vi "Update and Acknowledge InterruptBit HW.vi"(5 "Acknowledge?(True)":bool=TRUE, 7 "AcknPeriode":dbl, 8 "error in (no error)":errorcluster, 9 "current time":timestamp, 10 "InterruptBits":i32, 11 "BME_DG_Chnl in":refnum<class "BME_DG_Chnl.lvclass">) -> (0 "error out":errorcluster, 1 "ShotPeriode":dbl, 2 "ChnlBit":bool, 3 "BME_DG_Chnl out":refnum<class "BME_DG_Chnl.lvclass">)   [LabVIEW 2009, in "POLARIS BME DG.lvlib" / "BME_DG_Chnl.lvclass"]
uses:
  BME_DG_Chnl.lvclass
  BME_DG_Chnl.lvclass/BME_DG_Chnl.ctl
  POLARIS BME DG.lvlib
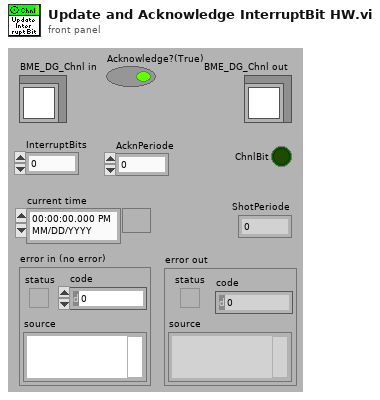
[diagram p1: front panel]
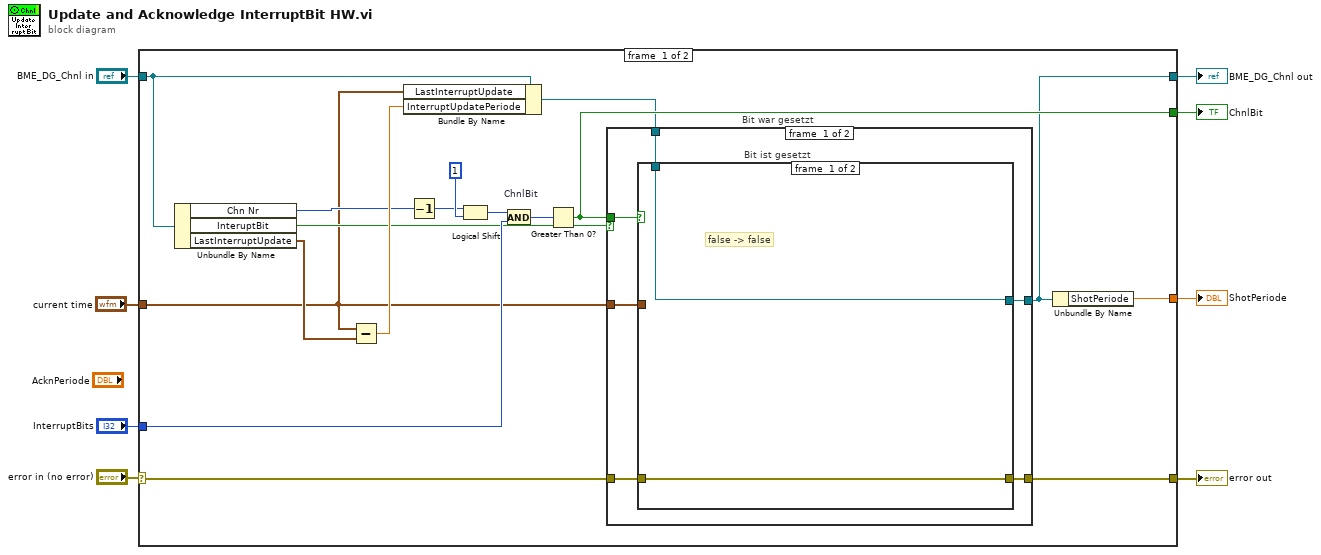
[diagram p0: block diagram]
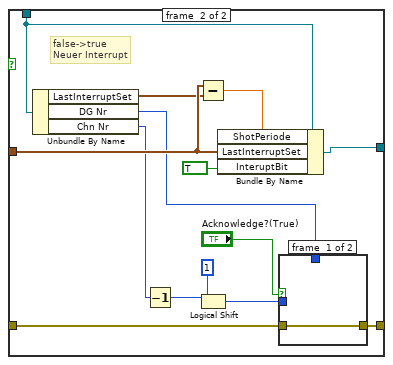
[diagram p2: hidden frame]
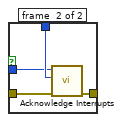
[diagram p3: hidden frame]
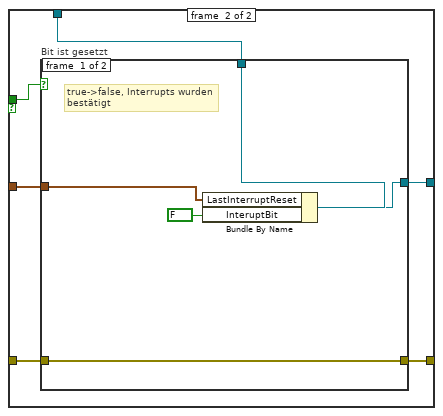
[diagram p4: hidden frame]
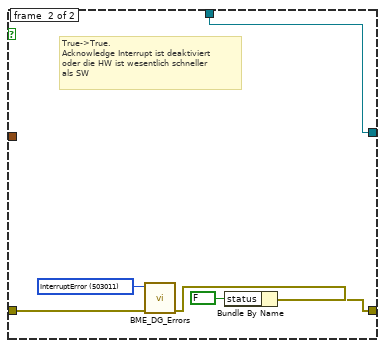
[diagram p5: hidden frame]
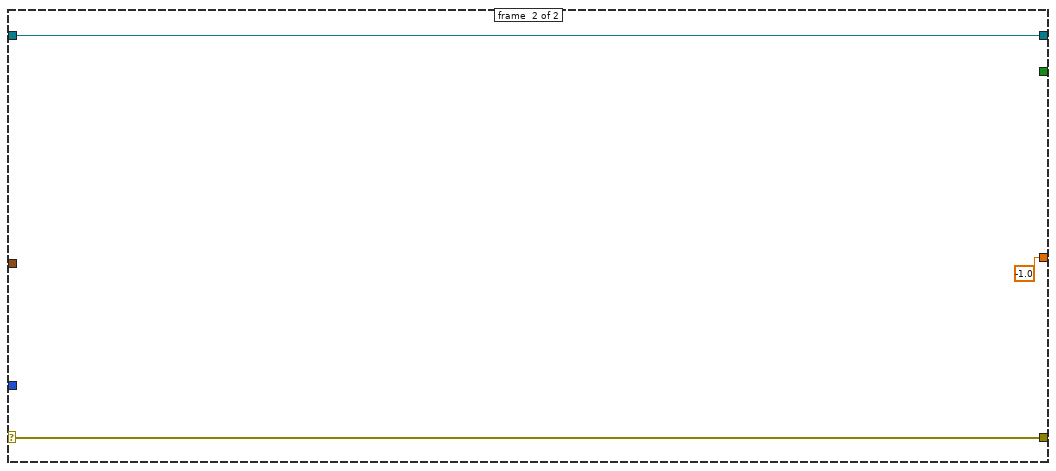
[diagram p6: hidden frame]
diagram:
  n1 = case shown="No Error" "error in (no error)" {
    selector: "error in (no error)" -> [w15 w70]
    tunnel: "BME_DG_Chnl in" -> [w13 w72]
    tunnel: "InterruptBits" -> [w22 _]
    tunnel: [w16 _] -> w6
    tunnel: [w11 w72] -> w5
    tunnel: "current time" -> [w12 _]
    tunnel: [w10 -1.0 ("f")] -> w3
    tunnel: [w14 w70] -> w1
    frame #0 {
      n2 = Unbundle By Name(w13) -> ("Chn Nr"=w18:i32, "InteruptBit"=w17:bool, "LastInterruptUpdate"=w20:timestamp)
      n3 = Subtract(x=w12, y=w20) -> (x-y=w19:dbl)
      n4 = Bundle By Name(cluster=w13, "LastInterruptUpdate"=w12, "InterruptUpdatePeriode"=w19) -> (w9:refnum<class "BME_DG_Chnl.lvclass">)
      n5 = Decrement(x=w18) -> (x-1=w24:i32)
      n6 = Logical Shift(y=w24, x=1) -> (x << y=w23:i32)
      n7 = And "ChnlBit"(x=w23, y=w22) -> (x .and. y?=w21:i32)
      n8 = Greater Than 0?(x=w21) -> (x > 0?=w16:bool)
      n9 = case "Bit war gesetzt" shown="False" w17 {
        tunnel: w16 -> [w31 w58]
        tunnel: w15 -> [w26 w57]
        tunnel: [w27 w56] -> w14
        tunnel: w9 -> [w30 w55]
        tunnel: w12 -> [w28 w54]
        tunnel: [w29 w53] -> w11
        frame #0 {
          n10 = case "Bit ist gesetzt" shown="True" w31 {
            tunnel: w30 -> [w33 w45]
            tunnel: [w33 w47] -> w29
            tunnel: w28 -> [_ w44]
            tunnel: [w32 w37] -> w27
            tunnel: w26 -> [w32 w38]
            frame #0 {
              # "false -> false"
            }
            frame #1 {
              # "false->true \nNeuer Interrupt"
              n11 = Unbundle By Name(w45) -> ("LastInterruptSet"=w43:timestamp, "DG Nr"=w36:i32, "Chn Nr"=w40:i32)
              n12 = Decrement(x=w40) -> (x-1=w41:i32)
              n13 = Subtract(x=w44, y=w43) -> (x-y=w42:dbl)
              n14 = Logical Shift(y=w41, x=1) -> (x << y=w35:i32)
              n15 = Bundle By Name(cluster=w45, "ShotPeriode"=w42, "LastInterruptSet"=w44, "InteruptBit"=TRUE) -> (w47:refnum<class "BME_DG_Chnl.lvclass">)
              n16 = case shown="True" "Acknowledge?(True)" {
                tunnel: w38 -> [w48 w52]
                tunnel: [w48 w51] -> w37
                tunnel: w36 -> [_ w50]
                tunnel: w35 -> [_ w49]
                frame #0 {
                }
                frame #1 {
                  n17 = call "Acknowledge Interrupts.vi"("error in (no error)"=w52, "DG Number"=w50, "Interrupt Ack"=w49) -> ("error out"=w51:errorcluster)  [unwired: 8 in]
                }
              }
            }
          }
        }
        frame #1 {
          n18 = case "Bit ist gesetzt" shown="False" w58 {
            tunnel: w57 -> [w59 w68]
            tunnel: [w59 w65] -> w56
            tunnel: w55 -> [w63 w64]
            tunnel: w54 -> [w61 _]
            tunnel: [w62 w64] -> w53
            frame #0 {
              # "true->false, Interrupts wurden\nbestätigt"
              n19 = Bundle By Name(cluster=w63, "LastInterruptReset"=w61, "InteruptBit"=FALSE) -> (w62:refnum<class "BME_DG_Chnl.lvclass">)
            }
            frame #1 {
              w69 = 503011 items=["Channel refers itself"=503001, "Deadloop"=503002, "Negative Delay"=503003, "Delay Card not found"=503004, "Channel not found"=503005, "Parse Error"=503006, "Not Supported"=503007, "Systen not found"=503008, "To much masters"=503009, "None master in Syterm"=503010, "InterruptError"=503011, "ChnlPeriodeWarning"=503012] ("error")
              # "True->True. \nAcknowledge Interrupt ist deaktiviert\noder die HW ist wesentlich schneller\nals SW"
              n20 = call "BME_DG_Errors.vi"("error in (no error)"=w68, "error"=w69) -> ("error out"=w67:errorcluster)  [unwired: 9 in]
              n21 = Bundle By Name(cluster=w67, "status"=FALSE) -> (w65:errorcluster)
            }
          }
        }
      }
      n22 = Unbundle By Name(w11) -> ("ShotPeriode"=w10:dbl)
    }
    frame #1 {
    }
  }
  "error out" <- w1
  "BME_DG_Chnl out" <- w5
  "ChnlBit" <- w6
  "ShotPeriode" <- w3
